vi "Update User Warning Dialog.vi"(8 "Error In":errorcluster, 11 "Warnings":T1[](array[typedef])) -> (0 "Error Out":errorcluster, 1 "Num Warnings":i32, 2 "User Warnings":T2[](array[typedef]), 3 "Warnings":T1[](array[typedef]))   [LabVIEW 2011, in "LMH-LINX.lvlib"]
uses:
  LMH-LINX.lvlib
  User Warning.ctl
  Target Compatibility Warnings.ctl
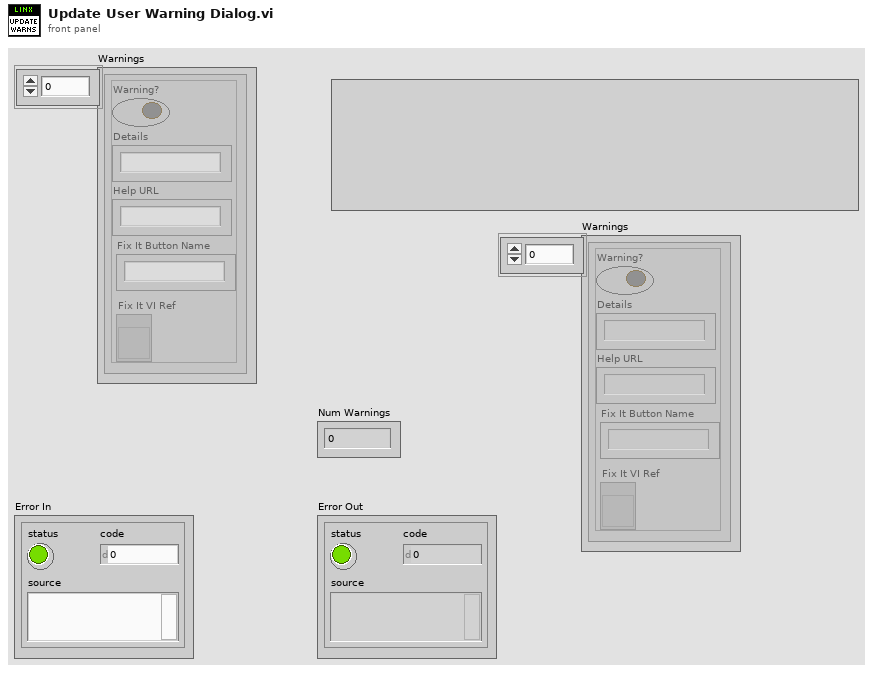
[diagram p1: front panel]
types:
  T1 = typedef "LMH-LINX.lvlib/Target Compatibility Warnings.ctl" = cluster{"Warning?":bool, "Details":string, "Help URL":string, "Fix It Button Name":string, "Fix It VI Ref":refnum<vi>}
  T2 = typedef "LMH-LINX.lvlib/User Warning.ctl" = cluster{"Details":string, "Status":string}
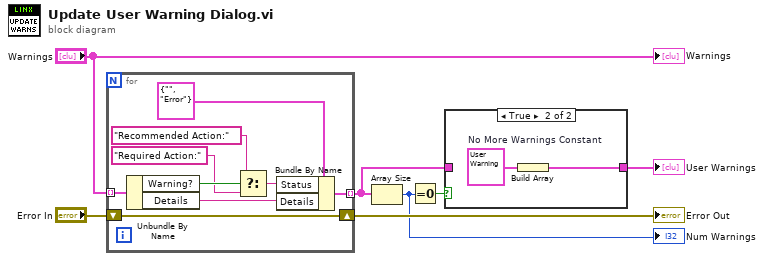
[diagram p0: block diagram]
diagram:
  n1 = for {
    tunnel: "Warnings" -> [w16] mode=indexing
    tunnel: [w9] -> w1 mode=indexing
    shift-right: [w8] -> w6
    shift-left: "Error In" -> [w8]
    n2 = Unbundle By Name(w16) -> ("Warning?"=w15:bool, "Details"=w11:string)
    n3 = Select(t="Recommended Action:", s=w15, f="Required Action:") -> (s? t:f=w12:string)
    n4 = Bundle By Name(cluster=T2 {"Details"="", "Status"="Error"} ("User Warning"), "Status"=w12, "Details"=w11) -> (w9:T2)
  }
  "Error Out" <- w6
  n5 = Array Size(array=w1) -> (size(s)=w4:i32)
  "Num Warnings" <- w4
  n6 = Equal To 0?(x=w4) -> (x = 0?=w3:bool)
  n7 = case shown="True" w3 {
    tunnel: [w17 w19] -> w2
    tunnel: w1 -> [w17 _]
    frame False {
    }
    frame True {
      w18 = T2 {"Details"="All issues have been resolved.  Click continue to continue the installation or cancel to quit.", "Status"="Status"}  # No More Warnings Constant
      n8 = Build Array(w18) -> (w19:T2[])
    }
  }
  "User Warnings" <- w2
  "Warnings" <- "Warnings"
